vi "Main Tclk.vi"() -> ()   [LabVIEW 2018] (continued)
                    n5601 = Bundle By Name(cluster=w4850, "X stig"=w4849, "Y stig"=w4848, "X aln"=w4847, "Y aln"=w4846, "WD (mm)"=w4845, "X tiles"=w4859, "Y tiles"=w4859, "dX (um)"=w4858, "dY (um)"=w4858, "X center (um)"=w4864, "Y center (um)"=w4864) -> (w4865:T26)
                    n5602 = local write "X shift (nm/image)"(w4864) -> ()
                    n5603 = local write "Y shift (nm/image)"(w4864) -> ()
                    n5604 = local write "SEM Scan Parameters"(w4865) -> ()
                  }
                }
              }
            }
          }
          event "SEM Options.Save": Value Change {
            n5605 = event-data() -> ("NewVal"=w4878:bool)  [unwired: 6 out]
            n5606 = case shown="False" w4878 {
              frame False {
                n5607 = local read "SEM Options"() -> (w4881:T27)
                n5608 = Bundle By Name(cluster=w4881, "Upload"=FALSE) -> (w4879:T27)
                n5609 = local write "SEM Options"(w4879) -> ()
              }
              frame True {
              }
            }
          }
          event "SEM Options.Upload": Value Change {
            n5610 = event-data() -> ("OldVal"=w4882:bool, "NewVal"=w4885:bool)  [unwired: 5 out]
            n5611 = local read "FIB"() -> (w4883:bool)
            n5612 = case shown="True" w4883 {
              tunnel: [TRUE ("T button?") w4887] -> w4884
              frame False {
              }
              frame True {
                n5613 = Two Button Dialog(message="Are you sure to change the  file upload settings?") -> (T button?=w4887:bool)  [unwired: 2 in]
              }
            }
            n5614 = case shown="True" w4884 {
              tunnel: w4885 -> [_ w4893]
              tunnel: w4882 -> [w4889 _]
              frame False {
                n5615 = local read "SEM Options"() -> (w4891:T27)
                n5616 = Bundle By Name(cluster=w4891, "Upload"=w4889) -> (w4890:T27)
                n5617 = local write "SEM Options"(w4890) -> ()
              }
              frame True {
                n5618 = case shown="True" w4893 {
                  frame False {
                  }
                  frame True {
                    n5619 = local read "SEM Options"() -> (w4900:T27)
                    n5620 = Bundle By Name(cluster=w4900, "Save"=TRUE ("Upload")) -> (w4898:T27)
                    n5621 = local write "SEM Options"(w4898) -> ()
                  }
                }
                n5622 = local read "Initial Options"() -> (w4894:T27)
                n5623 = Bundle By Name(cluster=w4894, "Upload"=w4893) -> (w4892:T27)
                n5624 = Select(t=T44."Enabled" ("Disabled"), s=w4893, f=T44."Disabled and Grayed Out" ("Disabled")) -> (s? t:f=w4897:T44)
                n5625 = local write "Initial Options"(w4892) -> ()
                n5626 = property on="Delete after upload" class="Bool (strict)"("DisabledEnum"=w4897) -> ()  [unwired: 2 in, 2 out]
              }
            }
          }
          event "SEM Options.8-bit": Value Change {
            n5627 = event-data() -> ("OldVal"=w4901:bool, "NewVal"=w4904:bool)  [unwired: 5 out]
            n5628 = local read "FIB"() -> (w4902:bool)
            n5629 = case shown="True" w4902 {
              tunnel: [TRUE ("T button?") w4906] -> w4903
              frame False {
              }
              frame True {
                n5630 = Two Button Dialog(message="Are you sure to change the  data type settings?") -> (T button?=w4906:bool)  [unwired: 2 in]
              }
            }
            n5631 = case shown="True" w4903 {
              tunnel: w4904 -> [_ w4912]
              tunnel: w4901 -> [w4908 _]
              frame False {
                n5632 = local read "SEM Options"() -> (w4910:T27)
                n5633 = Bundle By Name(cluster=w4910, "8-bit"=w4908) -> (w4909:T27)
                n5634 = local write "SEM Options"(w4909) -> ()
              }
              frame True {
                n5635 = local read "Initial Options"() -> (w4913:T27)
                n5636 = Bundle By Name(cluster=w4913, "8-bit"=w4912) -> (w4911:T27)
                n5637 = local write "Initial Options"(w4911) -> ()
              }
            }
          }
          event "Manual Upload": Value Change {
            n5638 = event-data() -> ()  [unwired: 7 out]
            n5639 = stacked-sequence {
              frame #0 {
                n5640 = local write "Manual Upload"(FALSE ("Manual Upload")) -> ()
              }
              frame #1 {
                n5641 = call "Enter sample ID and select options"() -> ("Delete after upload"=w4915:bool, "Sample ID"=w4916:string, "Next"=w4917:bool)  [unwired: 16 in, 1 out]
                n5642 = case shown="True" w4917 {
                  tunnel: w4916 -> [_ w4925]
                  tunnel: w4915 -> [_ w4924]
                  frame False {
                  }
                  frame True {
                    n5643 = local read "File Information"() -> (w4926:T31)
                    n5644 = Unbundle By Name(w4926) -> ("File path"=w4920:path)
                    n5645 = Path To String(path=w4920) -> (string=w4919:string)
                    n5646 = call "File dialog.vi"("Prompt"="Select SEM Files to Upload" ("prompt"), "Pattern"="*.dat" ("pattern label"), "InitialDirectory"=w4919) -> ("Cancelled"=w4918:bool, "FileNames"=w4923:string[])  [unwired: 7 in]
                    n5647 = case shown="False" w4918 {
                      tunnel: w4925 -> [w4929 _]
                      tunnel: w4924 -> [w4928 _]
                      tunnel: w4923 -> [w4927 _]
                      frame False {
                        n5648 = for {
                          tunnel: w4929 -> [w4933]
                          tunnel: w4928 -> [w4932]
                          tunnel: w4927 -> [w4930] mode=indexing
                          w4941 = "^" ("replace string (\"\")")
                          w4948 = T82 3 items=["no dialog", "OK message", "continue or stop message", "OK message + warnings", "continue/stop + warnings"] ("type of dialog (OK msg:1)")
                          n5649 = shared-variable ".\\Zeiss Library.lvlib\\Upload flags path"() -> (w4931:string)  [unwired: 1 in, 1 out]
                          n5650 = String To Path(string=w4931) -> (path=w4955:path)
                          n5651 = File/Directory Info(path=w4955) -> (path out=w4952:path, error out=w4954:errorcluster)  [unwired: 1 in, 5 out]
                          n5652 = Unbundle By Name(w4954) -> ("status"=w4953:bool)
                          n5653 = Search and Replace String(replace all?=TRUE ("replace all? (F)"), input string=w4930, search string="\\", replace string=w4941) -> (result string=w4940:string)  [unwired: 4 in, 3 out]
                          n5654 = case shown="True" w4953 {
                            tunnel: w4952 -> [w4956 w4958]
                            tunnel: [w4956 w4957] -> w4944
                            frame False {
                            }
                            frame True {
                              n5655 = Create Folder(path (use dialog)=w4958) -> (created path=w4957:path)  [unwired: 1 in, 3 out]
                            }
                          }
                          n5656 = Select(t="^delete" ("replace string (\"\")"), s=w4932, f="^keep" ("replace string (\"\")")) -> (s? t:f=w4935:string)
                          n5657 = Search and Replace String(input string=w4940, search string=":", replace string=w4941) -> (result string=w4937:string)  [unwired: 5 in, 3 out]
                          n5658 = Concatenate Strings(w4933, "^" ("string"), w4937, w4935) -> (w4945:string)
                          n5659 = Build Path(base path=w4944, name or relative path=w4945) -> (appended path=w4946:path)
                          n5660 = Open/Create/Replace File(file path (use dialog)=w4946, operation (0:open)=T49."replace or create") -> (refnum out=w4949:refnum<file>, error out=w4951:errorcluster)  [unwired: 1 in, 4 out]
                          n5661 = Close File(refnum=w4949, error in=w4951) -> (error out=w4950:errorcluster)  [unwired: 1 out]
                          n5662 = call <vilib>:"General Error Handler.vi"("type of dialog (OK msg:1)"=w4948, "error in (no error)"=w4950) -> ()  [unwired: 1 in, 13 out]
                        }
                      }
                      frame True {
                      }
                    }
                  }
                }
              }
            }
          }
          event "Focus index log": Mouse Down {
            n5663 = event-data() -> ("Coords"=w4968:T22)  [unwired: 8 out]
            n5664 = Unbundle By Name(w4968) -> ("Horizontal"=w4967:i32, "Vertical"=w4962:i32)
            n5665 = In Range and Coerce(upper limit=1200, x=w4967, lower limit=660 ("upper limit")) -> (In Range?=w4961:bool)  [unwired: 1 out]
            n5666 = In Range and Coerce(upper limit=366, x=w4962, lower limit=234 ("upper limit")) -> (In Range?=w4960:bool)  [unwired: 1 out]
            n5667 = And(x=w4961, y=w4960) -> (x .and. y?=w4959:bool)
            n5668 = case shown="True" w4959 {
              frame False {
              }
              frame True {
                n5669 = local read "FI toggle"() -> (w4969:bool)
                n5670 = case shown="False" w4969 {
                  frame False {
                    n5671 = local read "Log time array"() -> (w4972:u32[])
                    n5672 = local read "Focus index array"() -> (w4975:sgl[])
                    n5673 = local read "FI low limit array"() -> (w4971:sgl[])
                    n5674 = local write "FI toggle"(TRUE ("Delta X toggle")) -> ()
                    n5675 = property on="Focus index log" class="XYGraph (strict)"("YScale.NameLbl.Text"="Focus Index" ("Y Scale.Unit Label.Text")) -> ()  [unwired: 2 in, 2 out]
                    n5676 = Bundle("Log time array"=w4972, "Focus index array"=w4975) -> (w4974:T83)  [unwired: 1 in]
                    n5677 = Bundle("Log time array"=w4972, "FI low limit array"=w4971) -> (w4970:T84)  [unwired: 1 in]
                    n5678 = Build Array(w4974, w4970) -> (w4973:T85)
                    n5679 = local write "Focus index log"(w4973) -> ()
                  }
                  frame True {
                    n5680 = local read "Log time array"() -> (w4978:u32[])
                    n5681 = local read "FRC array"() -> (w4979:sgl[])
                    n5682 = local write "FI toggle"(FALSE ("Delta X toggle")) -> ()
                    n5683 = property on="Focus index log" class="XYGraph (strict)"("YScale.NameLbl.Text"="FRC resolution (nm)" ("Y Scale.Unit Label.Text")) -> ()  [unwired: 2 in, 2 out]
                    n5684 = Bundle("Log time array"=w4978, "FRC array"=w4979) -> (w4981:T86)  [unwired: 1 in]
                    n5685 = Build Array(w4981) -> (w4980:T87)
                    n5686 = local write "Focus index log"(w4980) -> ()
                  }
                }
              }
            }
          }
          event "Delta X log": Mouse Down {
            n5687 = event-data() -> ("Coords"=w4993:T22)  [unwired: 8 out]
            n5688 = Unbundle By Name(w4993) -> ("Horizontal"=w4992:i32, "Vertical"=w4987:i32)
            n5689 = In Range and Coerce(upper limit=1200, x=w4992, lower limit=660 ("upper limit")) -> (In Range?=w4986:bool)  [unwired: 1 out]
            n5690 = In Range and Coerce(upper limit=510, x=w4987, lower limit=378 ("upper limit")) -> (In Range?=w4985:bool)  [unwired: 1 out]
            n5691 = And(x=w4986, y=w4985) -> (x .and. y?=w4984:bool)
            n5692 = case shown="True" w4984 {
              frame False {
              }
              frame True {
                n5693 = local read "Delta X toggle"() -> (w4994:bool)
                n5694 = case shown="False" w4994 {
                  frame False {
                    n5695 = local read "Log time array"() -> (w4997:u32[])
                    n5696 = local read "Delta X array"() -> (w5002:sgl[])
                    n5697 = local read "Delta X stop limit array"() -> (w4995:sgl[])
                    n5698 = local write "Delta X toggle"(TRUE ("Delta X toggle")) -> ()
                    n5699 = property on="Delta X log" class="XYGraph (strict)"("YScale.NameLbl.Text"="Delta X (nm)" ("Y Scale.Unit Label.Text")) -> ()  [unwired: 2 in, 2 out]
                    n5700 = Negate(x=w4995) -> (-x=w4998:sgl[])
                    n5701 = Bundle("Log time array"=w4997, "Delta X array"=w5002) -> (w5001:T88)  [unwired: 1 in]
                    n5702 = Bundle("Log time array"=w4997, "Delta X stop limit array"=w4995) -> (w5000:T89)  [unwired: 1 in]
                    n5703 = Bundle("Log time array"=w4997, w4998) -> (w4996:cluster{"Log time array":u32[], sgl[]})  [unwired: 1 in]
                    n5704 = Build Array(w5001, w5000, w4996) -> (w4999:T39)
                    n5705 = local write "Delta X log"(w4999) -> ()
                  }
                  frame True {
                    n5706 = local read "Log time array"() -> (w5005:u32[])
                    n5707 = local read "Delta X sum array"() -> (w5006:sgl[])
                    n5708 = local write "Delta X toggle"(FALSE ("Delta X toggle")) -> ()
                    n5709 = property on="Delta X log" class="XYGraph (strict)"("YScale.NameLbl.Text"="Delta X sum (nm)" ("Y Scale.Unit Label.Text")) -> ()  [unwired: 2 in, 2 out]
                    n5710 = Bundle("Log time array"=w5005, "Delta X sum array"=w5006) -> (w5008:T90)  [unwired: 1 in]
                    n5711 = Build Array(w5008) -> (w5007:T91)
                    n5712 = local write "Delta X log"(w5007) -> ()
                  }
                }
              }
            }
          }
          event "Delta Y log": Mouse Down {
            n5713 = event-data() -> ("Coords"=w5011:T22)  [unwired: 8 out]
            n5714 = Unbundle By Name(w5011) -> ("Horizontal"=w5020:i32, "Vertical"=w5015:i32)
            n5715 = In Range and Coerce(upper limit=1200, x=w5020, lower limit=660 ("upper limit")) -> (In Range?=w5014:bool)  [unwired: 1 out]
            n5716 = In Range and Coerce(upper limit=654, x=w5015, lower limit=522 ("upper limit")) -> (In Range?=w5013:bool)  [unwired: 1 out]
            n5717 = And(x=w5014, y=w5013) -> (x .and. y?=w5012:bool)
            n5718 = case shown="True" w5012 {
              frame False {
              }
              frame True {
                n5719 = local read "Delta Y toggle"() -> (w5021:bool)
                n5720 = case shown="True" w5021 {
                  frame False {
                    n5721 = local read "Log time array"() -> (w5026:u32[])
                    n5722 = local read "Delta Y array"() -> (w5028:sgl[])
                    n5723 = local read "Delta X stop limit array"() -> (w5022:sgl[])
                    n5724 = local write "Delta Y toggle"(TRUE ("Delta X toggle")) -> ()
                    n5725 = property on="Delta Y log" class="XYGraph (strict)"("YScale.NameLbl.Text"="Delta Y (nm)" ("Y Scale.Unit Label.Text")) -> ()  [unwired: 2 in, 2 out]
                    n5726 = Negate(x=w5022) -> (-x=w5025:sgl[])
                    n5727 = Bundle("Log time array"=w5026, "Delta Y array"=w5028) -> (w5023:T92)  [unwired: 1 in]
                    n5728 = Bundle("Log time array"=w5026, "Delta X stop limit array"=w5022) -> (w5024:T89)  [unwired: 1 in]
                    n5729 = Bundle("Log time array"=w5026, w5025) -> (w5027:cluster{"Log time array":u32[], sgl[]})  [unwired: 1 in]
                    n5730 = Build Array(w5023, w5024, w5027) -> (w5029:T39)
                    n5731 = local write "Delta Y log"(w5029) -> ()
                  }
                  frame True {
                    n5732 = local read "Log time array"() -> (w5033:u32[])
                    n5733 = local read "Delta Y sum array"() -> (w5034:sgl[])
                    n5734 = local write "Delta Y toggle"(FALSE ("Delta X toggle")) -> ()
                    n5735 = property on="Delta Y log" class="XYGraph (strict)"("YScale.NameLbl.Text"="Delta Y sum (nm)" ("Y Scale.Unit Label.Text")) -> ()  [unwired: 2 in, 2 out]
                    n5736 = Bundle("Log time array"=w5033, "Delta Y sum array"=w5034) -> (w5032:T93)  [unwired: 1 in]
                    n5737 = Build Array(w5032) -> (w5035:T94)
                    n5738 = local write "Delta Y log"(w5035) -> ()
                  }
                }
              }
            }
          }
          event "Delta Z log": Mouse Down {
            n5739 = event-data() -> ("Coords"=w5040:T22, "PlatMods"=w5039:T77)  [unwired: 7 out]
            n5740 = Unbundle By Name(w5040) -> ("Horizontal"=w5049:i32, "Vertical"=w5044:i32)
            n5741 = Unbundle By Name(w5039) -> ("Shift"=w5038:bool)
            n5742 = In Range and Coerce(upper limit=1200, x=w5049, lower limit=660 ("upper limit")) -> (In Range?=w5043:bool)  [unwired: 1 out]
            n5743 = In Range and Coerce(upper limit=798, x=w5044, lower limit=666 ("upper limit")) -> (In Range?=w5042:bool)  [unwired: 1 out]
            n5744 = And(x=w5043, y=w5042) -> (x .and. y?=w5041:bool)
            n5745 = case shown="True" w5041 {
              tunnel: w5038 -> [_ w5050]
              frame False {
              }
              frame True {
                n5746 = local read "Delta Z mode"() -> (w5060:u8)
                n5747 = case shown="2" w5060 {
                  tunnel: [w5063 w5070 w5102] -> w5054
                  tunnel: w5050 -> [_ w5069 _]
                  frame 0, Default {
                    n5748 = local read "Delta Z mode"() -> (w5066:u8)
                    n5749 = local read "Log time array"() -> (w5068:u32[])
                    n5750 = local read "Delta Z array"() -> (w5063:sgl[])
                    n5751 = Increment(x=w5066) -> (x+1=w5065:u8)
                    n5752 = property on="Delta Z log" class="XYGraph (strict)"("YScale.NameLbl.Text"="Delta Z (nm)" ("Y Scale.Unit Label.Text")) -> ()  [unwired: 2 in, 2 out]
                    n5753 = Bundle("Log time array"=w5068, "Delta Z array"=w5063) -> (w5067:T95)  [unwired: 1 in]
                    n5754 = local write "Delta Z mode"(w5065) -> ()
                    n5755 = local write "Delta Z log"(w5067) -> ()
                  }
                  frame 1 {
                    n5756 = case shown="True" w5069 {
                      tunnel: [w5071 w5077] -> w5070
                      frame False {
                        n5757 = local read "Log time array"() -> (w5076:u32[])
                        n5758 = local read "Milling Z voltage array"() -> (w5071:sgl[])
                        n5759 = local read "Delta Z mode"() -> (w5074:u8)
                        n5760 = Increment(x=w5074) -> (x+1=w5073:u8)
                        n5761 = property on="Delta Z log" class="XYGraph (strict)"("YScale.NameLbl.Text"="Milling Z Voltage (V)" ("Y Scale.Unit Label.Text")) -> ()  [unwired: 2 in, 2 out]
                        n5762 = Bundle("Log time array"=w5076, "Milling Z voltage array"=w5071) -> (w5075:T96)  [unwired: 1 in]
                        n5763 = local write "Delta Z mode"(w5073) -> ()
                        n5764 = local write "Delta Z log"(w5075) -> ()
                      }
                      frame True {
                        n5765 = local read "Milling Z voltage array"() -> (w5089:sgl[])
                        n5766 = Array Size(array=w5089) -> (size(s)=w5088:i32)
                        n5767 = for {
                          N: w5088 -> [_]
                          tunnel: w5089 -> [w5100]
                          tunnel: [w5092] -> w5086 mode=indexing
                          tunnel: 100 ("sample length") -> [w5096]
                          i -> [w5095]
                          n5768 = Increment(x=w5095) -> (x+1=w5091:i32)
                          n5769 = Subtract(x=w5091, y=w5096) -> (x-y=w5099:i32)
                          n5770 = Max & Min(x=w5096, y=w5091) -> (min(x,y)=w5094:i32)  [unwired: 1 out]
                          n5771 = Array Subset(array=w5100, index=w5099, length=w5094) -> (w5098:sgl[])
                          n5772 = for {
                            N: w5094 -> [_]
                            tunnel: [w5101] -> w5093 mode=indexing
                            i -> [w5101]
                          }
                          n5773 = call <vilib>:"Linear Fit.vi"("Y"=w5098, "X"=w5093) -> ("slope"=w5097:dbl)  [unwired: 9 in, 4 out]
                          n5774 = To Single Precision Float(number=w5097) -> (single precision float=w5092:sgl)
                        }
                        n5775 = local read "FIB Scan Parameters"() -> (w5087:T32)
                        n5776 = local read "Milling para"() -> (w5084:T35)
                        n5777 = Unbundle By Name(w5087) -> ("Z size (V)"=w5085:dbl)
                        n5778 = Unbundle By Name(w5084) -> ("FIB FOV (um)"=w5082:sgl)
                        n5779 = To Single Precision Float(number=w5085) -> (single precision float=w5080:sgl)
                        n5780 = local read "Log time array"() -> (w5079:u32[])
                        n5781 = Divide(x=w5086, y=w5080) -> (x/y=w5083:sgl[])
                        n5782 = Compound Arithmetic op=MULTIPLY(w5083, w5082, sgl -1000.0 ("value")) -> (w5077:sgl[])
                        n5783 = Bundle("Log time array"=w5079, w5077) -> (w5078:cluster{"Log time array":u32[], sgl[]})  [unwired: 1 in]
                        n5784 = local write "Delta Z log"(w5078) -> ()
                      }
                    }
                  }
                  frame 2 {
                    n5785 = local read "Log time array"() -> (w5106:u32[])
                    n5786 = local read "Delta image array"() -> (w5102:sgl[])
                    n5787 = property on="Delta Z log" class="XYGraph (strict)"("YScale.NameLbl.Text"="Delta Image" ("Y Scale.Unit Label.Text")) -> ()  [unwired: 2 in, 2 out]
                    n5788 = Bundle("Log time array"=w5106, "Delta image array"=w5102) -> (w5105:T97)  [unwired: 1 in]
                    n5789 = local write "Delta Z mode"(u8 0 ("Delta Z mode")) -> ()
                    n5790 = local write "Delta Z log"(w5105) -> ()
                  }
                }
                n5791 = Array Subset(array=w5054, index=1) -> (w5053:sgl[])  [unwired: 1 in]
                n5792 = Array Size(array=w5053) -> (size(s)=w5051:i32)
                n5793 = call "Auto limits.vi"("Minimum half range"=0.2, "# of interquartile range or stdev"=1.5 ("# of sigma"), "Input array"=w5053) -> ("Low limit"=w5059:dbl, "High limit"=w5058:dbl)  [unwired: 6 in, 1 out]
                n5794 = Not Equal To 0?(x=w5051) -> (x != 0?=w5052:bool)
                n5795 = case shown="True" w5052 {
                  tunnel: w5058 -> [_ w5062]
                  tunnel: w5059 -> [_ w5061]
                  frame False {
                  }
                  frame True {
                    n5796 = property on="Delta Z log" class="XYGraph (strict)"("YScale.Maximum"=w5062) -> ()  [unwired: 2 in, 2 out]
                    n5797 = property on="Delta Z log" class="XYGraph (strict)"("YScale.Minimum"=w5061) -> ()  [unwired: 2 in, 2 out]
                  }
                }
              }
            }
          }
          event "Specimen I log": Mouse Down {
            n5798 = event-data() -> ("Coords"=w5108:T22)  [unwired: 8 out]
            n5799 = Unbundle By Name(w5108) -> ("Horizontal"=w5116:i32, "Vertical"=w5111:i32)
            n5800 = In Range and Coerce(upper limit=1200, x=w5116, lower limit=660 ("upper limit")) -> (In Range?=w5110:bool)  [unwired: 1 out]
            n5801 = In Range and Coerce(upper limit=654, x=w5111, lower limit=522 ("upper limit")) -> (In Range?=w5109:bool)  [unwired: 1 out]
            n5802 = And(x=w5110, y=w5109) -> (x .and. y?=w5107:bool)
            n5803 = case shown="True" w5107 {
              frame False {
              }
              frame True {
                n5804 = local read "Specimen current toggle"() -> (w5117:bool)
                n5805 = case shown="True" w5117 {
                  frame False {
                    n5806 = local read "Log time array"() -> (w5121:u32[])
                    n5807 = local read "Specimen I array"() -> (w5126:sgl[])
                    n5808 = local read "Specimen I high limit array"() -> (w5120:sgl[])
                    n5809 = local read "Specimen I low limit array"() -> (w5119:sgl[])
                    n5810 = property on="Specimen I log" class="XYGraph (strict)"("YScale.NameLbl.Text"="Specimen @ FIB (nA)" ("Y Scale.Unit Label.Text")) -> ()  [unwired: 2 in, 2 out]
                    n5811 = local write "Specimen current toggle"(TRUE ("Delta X toggle")) -> ()
                    n5812 = Bundle("Log time array"=w5121, "Specimen I array"=w5126) -> (w5123:T98)  [unwired: 1 in]
                    n5813 = Bundle("Log time array"=w5121, "Specimen I high limit array"=w5120) -> (w5124:T99)  [unwired: 1 in]
                    n5814 = Bundle("Log time array"=w5121, "Specimen I low limit array"=w5119) -> (w5118:T100)  [unwired: 1 in]
                    n5815 = Build Array(w5123, w5124, w5118) -> (w5122:T101)
                    n5816 = local write "Specimen I log"(w5122) -> ()
                  }
                  frame True {
                    n5817 = local read "Log time array"() -> (w5131:u32[])
                    n5818 = local read "SEM Specimen I array"() -> (w5135:sgl[])
                    n5819 = local read "SEM Specimen I high limit array"() -> (w5130:sgl[])
                    n5820 = local read "SEM Specimen I low limit array"() -> (w5129:sgl[])
                    n5821 = property on="Specimen I log" class="XYGraph (strict)"("YScale.NameLbl.Text"="Specimen @ SEM (nA)" ("Y Scale.Unit Label.Text")) -> ()  [unwired: 2 in, 2 out]
                    n5822 = local write "Specimen current toggle"(FALSE ("Delta X toggle")) -> ()
                    n5823 = Bundle("Log time array"=w5131, "SEM Specimen I array"=w5135) -> (w5133:T102)  [unwired: 1 in]
                    n5824 = Bundle("Log time array"=w5131, "SEM Specimen I high limit array"=w5130) -> (w5134:T103)  [unwired: 1 in]
                    n5825 = Bundle("Log time array"=w5131, "SEM Specimen I low limit array"=w5129) -> (w5128:T104)  [unwired: 1 in]
                    n5826 = Build Array(w5133, w5134, w5128) -> (w5132:T105)
                    n5827 = local write "Specimen I log"(w5132) -> ()
                  }
                }
              }
            }
          }
          event "Beam Dump log": Mouse Down {
            n5828 = event-data() -> ("Coords"=w5139:T22)  [unwired: 8 out]
            n5829 = Unbundle By Name(w5139) -> ("Horizontal"=w5147:i32, "Vertical"=w5142:i32)
            n5830 = In Range and Coerce(upper limit=1200, x=w5147, lower limit=660 ("upper limit")) -> (In Range?=w5141:bool)  [unwired: 1 out]
            n5831 = In Range and Coerce(upper limit=798, x=w5142, lower limit=666 ("upper limit")) -> (In Range?=w5140:bool)  [unwired: 1 out]
            n5832 = And(x=w5141, y=w5140) -> (x .and. y?=w5138:bool)
            n5833 = case shown="True" w5138 {
              frame False {
              }
              frame True {
                n5834 = local read "Beam dump display"() -> (w5148:u8)
                n5835 = case shown="0, Default" w5148 {
                  frame 0, Default {
                    w5158 = u8 1 items=["B.D.1", "B.D.2", "Mill"] ("Beam dump display")
                    n5836 = local read "Log time array"() -> (w5155:u32[])
                    n5837 = local read "Beam Dump 2 array"() -> (w5157:sgl[])
                    n5838 = local read "BD2 high limit array"() -> (w5150:sgl[])
                    n5839 = local read "BD2 low limit array"() -> (w5149:sgl[])
                    n5840 = local write "Beam dump display"(w5158) -> ()
                    n5841 = property on="Beam Dump log" class="XYGraph (strict)"("YScale.NameLbl.Text"="Beam Dump 2 (nA)" ("Y Scale.Unit Label.Text")) -> ()  [unwired: 2 in, 2 out]
                    n5842 = Bundle("Log time array"=w5155, "Beam Dump 2 array"=w5157) -> (w5154:T106)  [unwired: 1 in]
                    n5843 = Bundle("Log time array"=w5155, "BD2 high limit array"=w5150) -> (w5153:T107)  [unwired: 1 in]
                    n5844 = Bundle("Log time array"=w5155, "BD2 low limit array"=w5149) -> (w5152:T108)  [unwired: 1 in]
                    n5845 = Build Array(w5154, w5153, w5152) -> (w5151:T109)
                    n5846 = local write "Beam Dump log"(w5151) -> ()
                  }
                  frame 1 {
                    w5166 = u8 2 items=["B.D.1", "B.D.2", "Mill"] ("Beam dump display")
                    n5847 = local read "Log time array"() -> (w5160:u32[])
                    n5848 = local read "Milling I array"() -> (w5168:sgl[])
                    n5849 = local read "Milling I high limit array"() -> (w5163:sgl[])
                    n5850 = local read "Milling I low limit array"() -> (w5162:sgl[])
                    n5851 = local write "Beam dump display"(w5166) -> ()
                    n5852 = property on="Beam Dump log" class="XYGraph (strict)"("YScale.NameLbl.Text"="Mill Current (nA)" ("Y Scale.Unit Label.Text")) -> ()  [unwired: 2 in, 2 out]
                    n5853 = Bundle("Log time array"=w5160, "Milling I array"=w5168) -> (w5161:T110)  [unwired: 1 in]
                    n5854 = Bundle("Log time array"=w5160, "Milling I high limit array"=w5163) -> (w5165:T111)  [unwired: 1 in]
                    n5855 = Bundle("Log time array"=w5160, "Milling I low limit array"=w5162) -> (w5164:T112)  [unwired: 1 in]
                    n5856 = Build Array(w5161, w5165, w5164) -> (w5159:T113)
                    n5857 = local write "Beam Dump log"(w5159) -> ()
                  }
                  frame 2 {
                    w5178 = u8 0 items=["B.D.1", "B.D.2", "Mill"] ("Beam dump display")
                    n5858 = local read "Log time array"() -> (w5170:u32[])
                    n5859 = local read "Beam Dump 1 array"() -> (w5177:sgl[])
                    n5860 = local read "BD1 high limit array"() -> (w5174:sgl[])
                    n5861 = local read "BD1 low limit array"() -> (w5173:sgl[])
                    n5862 = local write "Beam dump display"(w5178) -> ()
                    n5863 = property on="Beam Dump log" class="XYGraph (strict)"("YScale.NameLbl.Text"="Beam Dump 1 (nA)" ("Y Scale.Unit Label.Text")) -> ()  [unwired: 2 in, 2 out]
                    n5864 = Bundle("Log time array"=w5170, "Beam Dump 1 array"=w5177) -> (w5172:T114)  [unwired: 1 in]
                    n5865 = Bundle("Log time array"=w5170, "BD1 high limit array"=w5174) -> (w5171:T115)  [unwired: 1 in]
                    n5866 = Bundle("Log time array"=w5170, "BD1 low limit array"=w5173) -> (w5175:T116)  [unwired: 1 in]
                    n5867 = Build Array(w5172, w5171, w5175) -> (w5169:T117)
                    n5868 = local write "Beam Dump log"(w5169) -> ()
                  }
                }
              }
            }
          }
          event "Request to reheat": Value Change {
            n5869 = event-data() -> ("NewVal"=w5179:bool)  [unwired: 6 out]
            n5870 = case shown="True" w5179 {
              frame False {
              }
              frame True {
                n5871 = stacked-sequence {
                  frame #0 {
                    n5872 = Two Button Dialog(message="Reheat FIB source?") -> (T button?=w5180:bool)  [unwired: 2 in]
                    n5873 = local write "Start Reheat"(w5180) -> ()
                  }
                  frame #1 {
                    n5874 = local write "Request to reheat"(FALSE ("Request to reheat")) -> ()
                  }
                }
              }
            }
          }
          event "Request to stop reheat": Value Change {
            n5875 = event-data() -> ("NewVal"=w5183:bool)  [unwired: 6 out]
            n5876 = case shown="True" w5183 {
              frame False {
              }
              frame True {
                n5877 = stacked-sequence {
                  frame #0 {
                    n5878 = Two Button Dialog(message="Stop FIB Reheat?") -> (T button?=w5184:bool)  [unwired: 2 in]
                    n5879 = local write "Stop Reheat"(w5184) -> ()
                  }
                  frame #1 {
                    n5880 = local write "Request to stop reheat"(FALSE ("Request to reheat")) -> ()
                  }
                }
              }
            }
          }
          event "Open FIB gun valve": Value Change {
            n5881 = event-data() -> ("OldVal"=w5187:bool, "NewVal"=w5188:bool)  [unwired: 5 out]
            n5882 = case shown="True" w5188 {
              tunnel: w5187 -> [w5189 w5195]
              frame False {
                n5883 = stacked-sequence {
                  tunnel: w5189 -> [w5190 _]
                  frame #0 {
                    n5884 = local write "Open FIB gun valve"(w5190) -> ()
                  }
                  frame #1 {
                    n5885 = Two Button Dialog(message="Close FIB Gun Valve?") -> (T button?=w5191:bool)  [unwired: 2 in]
                    n5886 = case shown="True" w5191 {
                      frame False {
                      }
                      frame True {
                        n5887 = local read "Api"() -> (w5194:refnum<k7>)
                        n5888 = call "SmartSEM Remote API FIB Gun Valve.vi"("FIB Gun Valve"=enum16{"Close", "Open"}."Close", "ActiveX Container"=w5194) -> ()  [unwired: 8 in, 2 out]
                      }
                    }
                  }
                }
              }
              frame True {
                n5889 = stacked-sequence {
                  tunnel: w5195 -> [w5196 _]
                  frame #0 {
                    n5890 = local write "Open FIB gun valve"(w5196) -> ()
                  }
                  frame #1 {
                    n5891 = Two Button Dialog(message="Open FIB Gun Valve?") -> (T button?=w5197:bool)  [unwired: 2 in]
                    n5892 = case shown="True" w5197 {
                      frame False {
                      }
                      frame True {
                        n5893 = local read "Api"() -> (w5200:refnum<k7>)
                        n5894 = call "SmartSEM Remote API FIB Gun Valve.vi"("FIB Gun Valve"=enum16{"Close", "Open"}."Open", "ActiveX Container"=w5200) -> ()  [unwired: 8 in, 2 out]
                      }
                    }
                  }
                }
              }
            }
          }
          event "Turn on FIB gun": Value Change {
            n5895 = event-data() -> ("NewVal"=w5202:bool)  [unwired: 6 out]
            n5896 = local read "Machine Type"() -> (w5201:u8)
            n5897 = case shown="True" w5202 {
              tunnel: w5201 -> [_ w5203]
              frame False {
              }
              frame True {
                n5898 = case shown="2" w5203 {
                  frame 0 {
                    n5899 = stacked-sequence {
                      frame #0 {
                        n5900 = local read "HV Data Output"() -> (w5206:T18)
                        n5901 = Unbundle By Name(w5206) -> ("Tip Lifetime (hr)"=w5205:sgl)
                        n5902 = Equal To 0?(x=w5205) -> (x = 0?=w5204:bool)
                        n5903 = case shown="True" w5204 {
                          frame False {
                          }
                          frame True {
                            n5904 = for {
                              N: 5 -> [_]
                              stop <- w5209 stop-if-true
                              n5905 = Wait Until Next ms Multiple(millisecond multiple=u32 100) -> ()  [unwired: 1 out]
                              n5906 = call "Read FIB Log Files.vi"("Log file path"=path "C:/Program Files (x86)/FEI Company/BDS/LogHVData.log") -> ("HV Data Output"=w5226:T118)  [unwired: 9 in, 1 out]
                              n5907 = Unbundle By Name(w5226) -> ("Filament (A)"=w5225:sgl, "Acclerator (V)"=w5224:sgl, "AccI (uA)"=w5223:sgl, "Extractor (V)"=w5222:sgl, "Emission (uA)"=w5221:sgl, "Suppressor (V)"=w5220:sgl, "SuppI (uA)"=w5219:sgl, "Lens1 (V)"=w5218:sgl, "Lens1I (uA)"=w5217:sgl, "Lens2 (V)"=w5216:sgl, "Lens2I (uA)"=w5215:sgl, "Tip Lifetime (hr)"=w5212:sgl)
                              n5908 = local write "HV Data Output"(w5226) -> ()
                              n5909 = Build Array(w5225, w5224, w5223, w5222, w5221, w5220, w5219, w5218, w5217, w5216, w5215, w5212) -> (w5214:sgl[])
                              n5910 = Add Array Elements(numeric array=w5214) -> (sum=w5213:sgl)
                              n5911 = Not Equal To 0?(x=w5213) -> (x != 0?=w5210:bool)
                              n5912 = Not Equal To 0?(x=w5212) -> (x != 0?=w5211:bool)
                              n5913 = Or(x=w5210, y=w5211) -> (x .or. y?=w5209:bool)
                            }
                          }
                        }
                      }
                      frame #1 {
                        n5914 = Two Button Dialog(message="Turn FIB Gun on without Reheat?") -> (T button?=w5228:bool)  [unwired: 2 in]
                        "Turn FIB Gun on" <- w5228
                        n5915 = local write "Start Reheat"(w5228) -> ()
                      }
                      frame #2 {
                        n5916 = local write "Turn on FIB gun"(FALSE ("Request to reheat")) -> ()
                      }
                    }
                  }
                  frame 1, Default {
                  }
                  frame 2 {
                    n5917 = Two Button Dialog(message="Turn FIB Gun on without Reheat?") -> (T button?=w5231:bool)  [unwired: 2 in]
                    n5918 = case shown="True" w5231 {
                      frame False {
                      }
                      frame True {
                        n5919 = local read "Api"() -> (w5235:refnum<k7>)
                        n5920 = invoke class="_EMApi" method="Execute"(reference=w5235, "lpszCommand"="CMD_FIB_GUN_ON") -> ()  [unwired: 2 in, 4 out]
                        n5921 = property on="Turn off FIB gun" class="Bool (strict)"("DisabledEnum"=T44."Enabled" ("Disabled")) -> ()  [unwired: 2 in, 2 out]
                      }
                    }
                  }
                }
              }
            }
          }
          event "Turn off FIB gun": Value Change {
            n5922 = event-data() -> ("NewVal"=w5236:bool)  [unwired: 6 out]
            n5923 = case shown="True" w5236 {
              frame False {
              }
              frame True {
                n5924 = Two Button Dialog(message="Turn FIB Gun off?") -> (T button?=w5237:bool)  [unwired: 2 in]
                n5925 = case shown="True" w5237 {
                  frame False {
                    n5926 = local write "Turn off FIB gun"(FALSE ("Turn off FIB gun")) -> ()
                  }
                  frame True {
                    n5927 = local read "Api"() -> (w5241:refnum<k7>)
                    n5928 = invoke class="_EMApi" method="Execute"(reference=w5241, "lpszCommand"="CMD_FIB_GUN_OFF") -> ()  [unwired: 2 in, 4 out]
                  }
                }
              }
            }
          }
          event "Turn FIB gun standby": Value Change {
            n5929 = event-data() -> ("NewVal"=w5242:bool)  [unwired: 6 out]
            n5930 = case shown="True" w5242 {
              frame False {
              }
              frame True {
                n5931 = Two Button Dialog(message="Put FIB Gun to Standby?") -> (T button?=w5243:bool)  [unwired: 2 in]
                n5932 = case shown="True" w5243 {
                  frame False {
                    n5933 = local write "Turn FIB gun standby"(FALSE ("Turn off FIB gun")) -> ()
                  }
                  frame True {
                    n5934 = local read "Api"() -> (w5247:refnum<k7>)
                    n5935 = invoke class="_EMApi" method="Execute"(reference=w5247, "lpszCommand"="CMD_FIB_GUN_STANDBY") -> ()  [unwired: 2 in, 4 out]
                  }
                }
              }
            }
          }
          event "Get V/I slope": Value Change {
            n5936 = event-data() -> ("NewVal"=w5248:bool)  [unwired: 6 out]
            n5937 = case shown="True" w5248 {
              frame False {
              }
              frame True {
                n5938 = Two Button Dialog(message="Check FIB source V/I slope?") -> (T button?=w5249:bool)  [unwired: 2 in]
                n5939 = case shown="True" w5249 {
                  frame False {
                    n5940 = local write "Get V/I slope"(FALSE ("Turn off FIB gun")) -> ()
                  }
                  frame True {
                    n5941 = local read "Api"() -> (w5254:refnum<k7>)
                    n5942 = local write "Get V/I slope"(FALSE ("Turn off FIB gun")) -> ()
                    n5943 = call "SmartSEM Remote API FIB VI slope.vi"("ActiveX Container"=w5254) -> ("V/I slope"=→"FIB V/I slope":sgl)  [unwired: 8 in, 2 out]
                  }
                }
              }
            }
          }
          event "Email Alert Recipients": Value Change {
            n5944 = event-data() -> ("NewVal"=w5256:string[])  [unwired: 6 out]
            n5945 = local read "FIB"() -> (w5255:bool)
            n5946 = case shown="True" w5255 {
              tunnel: w5256 -> [_ w5257]
              frame False {
              }
              frame True {
                n5947 = local read "Email recipents file"() -> (w5263:path)
                n5948 = Open/Create/Replace File(file path (use dialog)=w5263, operation (0:open)=T49."replace or create") -> (refnum out=w5262:refnum<file>, error out=w5261:errorcluster)  [unwired: 4 in, 1 out]
                n5949 = Write to Text File(file (use dialog)=w5262, text=w5257, error in=w5261) -> (refnum out=w5260:refnum<file>, error out=w5259:errorcluster)  [unwired: 1 in, 1 out]
                n5950 = Close File(refnum=w5260, error in=w5259) -> ()  [unwired: 2 out]
              }
            }
          }
          event "Focus Index Options.X Grids": Mouse Down; "Focus Index Options.X Grids": Value Change {
            n5951 = event-data() -> ()  [unwired: 5 out]
            n5952 = disable-structure shown="Disabled" {
              frame Disabled {
                n5953 = local read "Focus Index Options"() -> (w5276:T28)
                n5954 = Unbundle By Name(w5276) -> ("Focus Index primary grid center"=w5268:bool, "Primary X index"=w5277:u8[][], "Y Grids"=w5278:u8[][], "Primary Y index"=w5279:u8[][])  [unwired: 1 out]
                n5955 = local read "SEM Scan Parameters"() -> (w5284:T26)
                n5956 = Unbundle By Name(w5276) -> ("X Grids"=w5280:u8[][])
                n5957 = Unbundle By Name(w5284) -> ("X tiles"=w5283:u8, "Y tiles"=w5282:u8)
                n5958 = Select(t=2.0 ("Data Entry Limits:Increment"), s=w5268, f=1.0 ("Data Entry Limits:Increment")) -> (s? t:f=w5270:dbl)
                n5959 = call "2D array edit.vi"("min"=u8 1 ("x"), "max"=u8 100 ("x"), "Set boundaries"=TRUE ("Set boundary"), "Data Entry Limits:Increment"=w5270, "Display Format:Precision"=u8 0, "Rows"=w5282, "Columns"=w5283, "Caption.Text"="X Grids", "Input array"=w5280) -> ("Output array"=w5275:sgl[][])  [unwired: 2 in]
                n5960 = case shown="False" w5268 {
                  tunnel: w5275 -> [w5291 w5313]
                  tunnel: w5277 -> [w5290 _]
                  tunnel: w5278 -> [w5289 w5312]
                  tunnel: w5279 -> [w5288 _]
                  tunnel: w5276 -> [w5287 w5311]
                  frame False {
                    n5961 = for {
                      tunnel: w5291 -> [w5303] mode=indexing
                      tunnel: w5290 -> [w5302] mode=indexing
                      tunnel: [w5301] -> w5295 mode=indexing
                      tunnel: w5289 -> [w5300] mode=indexing
                      tunnel: w5288 -> [w5299] mode=indexing
                      tunnel: [w5298] -> w5294 mode=indexing
                      tunnel: u8 1 ("x") -> [w5297]
                      tunnel: [w5296] -> w5286 mode=indexing
                      n5962 = for {
                        tunnel: w5303 -> [w5304] mode=indexing
                        tunnel: w5302 -> [w5310] mode=indexing
                        tunnel: [w5309] -> w5301 mode=indexing
                        tunnel: w5300 -> [w5308] mode=indexing
                        tunnel: w5299 -> [w5307] mode=indexing
                        tunnel: [w5306] -> w5298 mode=indexing
                        tunnel: w5297 -> [w5305]
                        tunnel: [w5304] -> w5296 mode=indexing
                        n5963 = In Range and Coerce(upper limit=w5304, x=w5310, lower limit=w5305) -> (coerced(x)=w5309:sgl)  [unwired: 1 out]
                        n5964 = In Range and Coerce(upper limit=w5308, x=w5307, lower limit=w5305) -> (coerced(x)=w5306:u8)  [unwired: 1 out]
                      }
                    }
                    n5965 = Bundle By Name(cluster=w5287, "X Grids"=w5286, "Primary X index"=w5295, "Primary Y index"=w5294) -> (w5293:T28)
                    n5966 = local write "Focus Index Options"(w5293) -> ()
                  }
                  frame True {
                    n5967 = for {
                      tunnel: w5313 -> [w5324] mode=indexing
                      tunnel: w5312 -> [w5323] mode=indexing
                      tunnel: [w5322] -> w5317 mode=indexing
                      tunnel: [w5321] -> w5316 mode=indexing
                      tunnel: [w5320] -> w5315 mode=indexing
                      tunnel: [w5319] -> w5314 mode=indexing
                      n5968 = for {
                        tunnel: w5324 -> [w5330] mode=indexing
                        tunnel: w5323 -> [w5329] mode=indexing
                        tunnel: [w5328] -> w5322 mode=indexing
                        tunnel: [w5327] -> w5321 mode=indexing
                        tunnel: [w5326] -> w5320 mode=indexing
                        tunnel: [w5325] -> w5319 mode=indexing
                        n5969 = To Single Precision Float(number=w5330) -> (single precision float=w5333:sgl)
                        n5970 = To Single Precision Float(number=w5329) -> (single precision float=w5332:sgl)
                        n5971 = expression code="x/2"(w5333) -> (w5334:sgl)
                        n5972 = expression code="x/2"(w5332) -> (w5331:sgl)
                        n5973 = Round Toward +Infinity(x=w5334) -> (ceil(x): smallest int >= x=w5327:sgl)
                        n5974 = Round Toward +Infinity(x=w5331) -> (ceil(x): smallest int >= x=w5325:sgl)
                        n5975 = expression code="x*2-1"(w5327) -> (w5328:sgl)
                        n5976 = expression code="x*2-1"(w5325) -> (w5326:sgl)
                      }
                    }
                    n5977 = Bundle By Name(cluster=w5311, "X Grids"=w5317, "Primary X index"=w5316, "Y Grids"=w5315, "Primary Y index"=w5314) -> (w5318:T28)
                    n5978 = local write "Focus Index Options"(w5318) -> ()
                  }
                }
              }
              frame Enabled {
              }
            }
            n5979 = local write "FI array for stop limit"(sgl[] [] ("FI array for stop limit")) -> ()
            n5980 = local read "Focus Index Options"() -> (w5264:T28)
            n5981 = local read "SEM Scan Parameters"() -> (w5265:T26)
            n5982 = call "Focus Grid Chooser.vi"("SEM Scan Parameters"=w5265, "Focus Index Options"=w5264) -> ("Focus Index Options Out"=w5266:T28)  [unwired: 9 in]
            n5983 = local write "Focus Index Options"(w5266) -> ()
          }
          event "Focus Index Options.Y Grids": Mouse Down; "Focus Index Options.Y Grids": Value Change {
            n5984 = event-data() -> ()  [unwired: 5 out]
            n5985 = disable-structure shown="Disabled" {
              frame Disabled {
                n5986 = local read "Focus Index Options"() -> (w5348:T28)
                n5987 = Unbundle By Name(w5348) -> ("Focus Index primary grid center"=w5341:bool, "X Grids"=w5340:u8[][], "Primary X index"=w5349:u8[][], "Primary Y index"=w5350:u8[][])  [unwired: 1 out]
                n5988 = local read "SEM Scan Parameters"() -> (w5355:T26)
                n5989 = Unbundle By Name(w5348) -> ("Y Grids"=w5351:u8[][])
                n5990 = Unbundle By Name(w5355) -> ("X tiles"=w5354:u8, "Y tiles"=w5353:u8)
                n5991 = Select(t=2.0 ("Data Entry Limits:Increment"), s=w5341, f=1.0 ("Data Entry Limits:Increment")) -> (s? t:f=w5343:dbl)
                n5992 = call "2D array edit.vi"("min"=u8 1 ("x"), "max"=u8 100 ("x"), "Set boundaries"=TRUE ("Set boundary"), "Data Entry Limits:Increment"=w5343, "Display Format:Precision"=u8 0, "Rows"=w5353, "Columns"=w5354, "Caption.Text"="Y Grids", "Input array"=w5351) -> ("Output array"=w5339:sgl[][])  [unwired: 2 in]
                n5993 = case shown="False" w5341 {
                  tunnel: w5340 -> [w5362 w5384]
                  tunnel: w5349 -> [w5361 _]
                  tunnel: w5339 -> [w5360 w5383]
                  tunnel: w5350 -> [w5359 _]
                  tunnel: w5348 -> [w5358 w5382]
                  frame False {
                    n5994 = for {
